vi "Init Verbose Message.vi"(5 "Verbose Message":refnum<class "TestManagerMsg.Verbose.lvclass">, 7 "overwrite?":bool=TRUE, 9 "explanation":string, 10 "self-id":string, 11 "owner-id":string) -> (3 "Message":refnum<class "TestManagerMsg.lvclass">)   [LabVIEW 2020, in "Caraya.lvlib" / "TestManagerMsg.Verbose.lvclass"]
uses:
  TestManagerMsg.Verbose.lvclass
  C:/projects/caraya/src/classes/Test Manager Message/TestManagerMsg.lvclass
  Test Manager Message/TestManagerMsg.lvclass
  TestManagerMsg.Verbose.lvclass/TestManagerMsg.Verbose.ctl
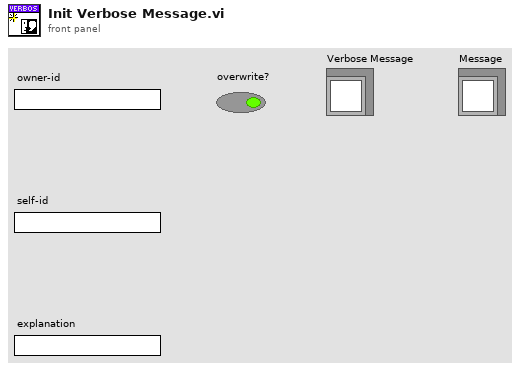
[diagram p1: front panel]
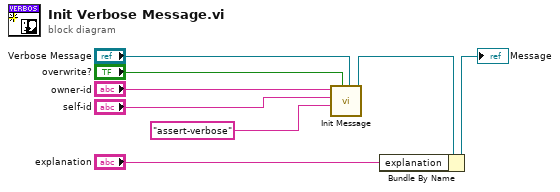
[diagram p0: block diagram]
diagram:
  n1 = call "Init Message.vi"("TestManagerMsg"="Verbose Message", "overwrite?"="overwrite?", "key"="assert-verbose", "self-id"="self-id", "owner-id"="owner-id") -> ("Message"=w6:refnum<class "TestManagerMsg.Verbose.lvclass">)  [unwired: 6 in]
  n2 = Bundle By Name(cluster=w6, "explanation"="explanation") -> (→"Message":refnum<class "TestManagerMsg.Verbose.lvclass">)
